vi "Init.vi"(3 "Container State":T3, 4 "Previous State":variant, 5 "Previous Version":T2) -> (2 "Current State":T1)   [LabVIEW 2020, in "WebView2 Control.xctl"]
uses:
  WebView2 Control.xctl
  Webview2 Lib/WebView2 Control Object/WebView2 Control.lvclass
  State.ctl
  <vilib>/_xctls/Container State.ctl
  <vilib>/_xctls/XControlSupport.lvlib
  <vilib>/_xctls/Version.ctl
panel:
  in  "Default Indicator State":T1
  in  "Default Control State":T1
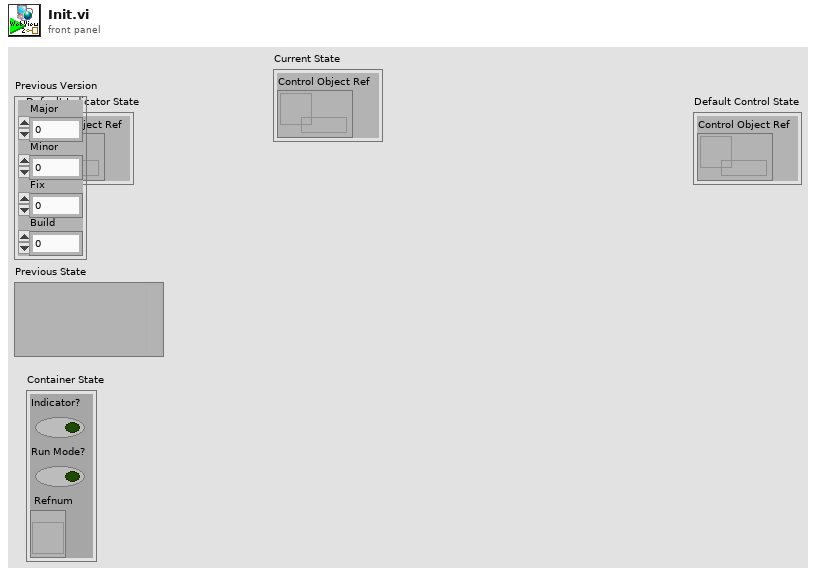
[diagram p1: front panel]
types:
  T1 = typedef "WebView2 Control.xctl/State.ctl" = cluster{"Control Object Ref":refnum<data-value>}
  T2 = typedef "XControlSupport.lvlib/Version.ctl" = cluster{"Major":u16, "Minor":u16, "Fix":u16, "Build":u16}
  T3 = typedef "XControlSupport.lvlib/Container State.ctl" = cluster{"Indicator?":bool, "Run Mode?":bool, " Refnum":refnum<vi>}
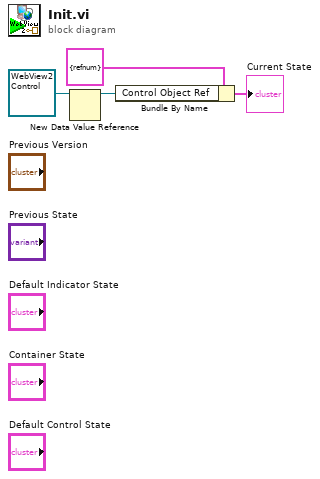
[diagram p0: block diagram]
diagram:
  n1 = New Data Value Reference(data value=refnum<class "WebView2 Control.lvclass"> refnum ("WebView2 Control")) -> (data value reference=w1:refnum<data-value>)  [unwired: 1 in, 1 out]
  n2 = Bundle By Name(cluster=T1 {"Control Object Ref"=refnum} ("Default Control State"), "Control Object Ref"=w1) -> (→"Current State":T1)
